vi "Add Error.vi"(8 "error in (no error)":errorcluster, 9 "String to Append":string, 10 "Error":T1, 11 "Insert Error":bool=TRUE) -> (0 "error out":errorcluster)   [LabVIEW 2021, in "ChannelCommon.lvlib"]
uses:
  ChannelCommon.lvlib
  typedef/Errors.ctl
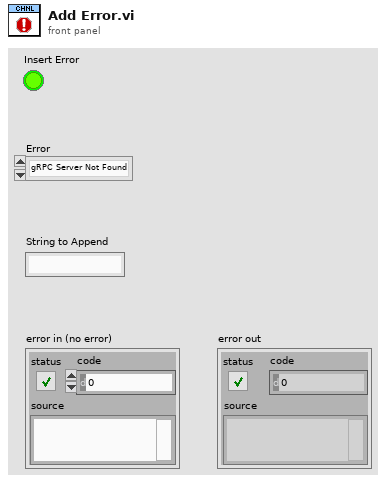
[diagram p1: front panel]
types:
  T1 = typedef "ChannelCommon.lvlib/Errors.ctl" = enum16{"gRPC Server Not Found", "Duplicate Channel", "Missing Channel", "Incorrect Type", "Flatten Error", "Unflatten Data", "Channel Length", "Plugin Connection", "gRPC Server Connection", "FIFO Unflatten", "Required Override", "Remove Not Found", "Multi Sub Not Supported", "Primary Already Connected", "Backpressure Not Supported", "Unable to Increase Buffer", "Data too Large"}
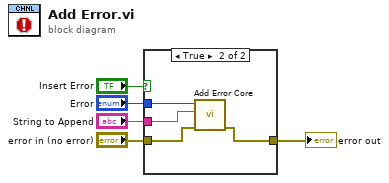
[diagram p0: block diagram]
diagram:
  n1 = case shown="True" "Insert Error" {
    tunnel: [w6 w7] -> w4
    tunnel: "error in (no error)" -> [w6 w8]
    tunnel: "Error" -> [_ w10]
    tunnel: "String to Append" -> [_ w9]
    frame False {
    }
    frame True {
      n2 = call "Add Error Core.vi"("error in (no error)"=w8, "String to Append"=w9, "Error"=w10) -> ("error out"=w7:errorcluster)  [unwired: 8 in]
    }
  }
  "error out" <- w4
